vi "AMI_SetVoltage.vi"(6 "error in (no error)":errorcluster, 7 "Index":i8) -> (0 "error out":errorcluster, 2 "resulting string 1":string="        Set Temperatura 4.2K at 20K/min, FastSettle", 3 "Cancelled?":bool)   [LabVIEW 2017]
doc: "Use this template to create a dialog box. This template polls the state of the buttons on the front panel and does not use events. Use the Dialog Using Events template (not available in Base package) to create a dialog box with event handling."
panel:
  in  "Wait stability":bool=TRUE
  in  "Rate (V/min)":dbl=20.0
  in  "Voltage (V)":dbl=5.0
  in  "Cancel":bool
  in  "OK":bool
  # "SET VOLTAGE"
  # "Enero 2023 V1.3  a-sslcdms"
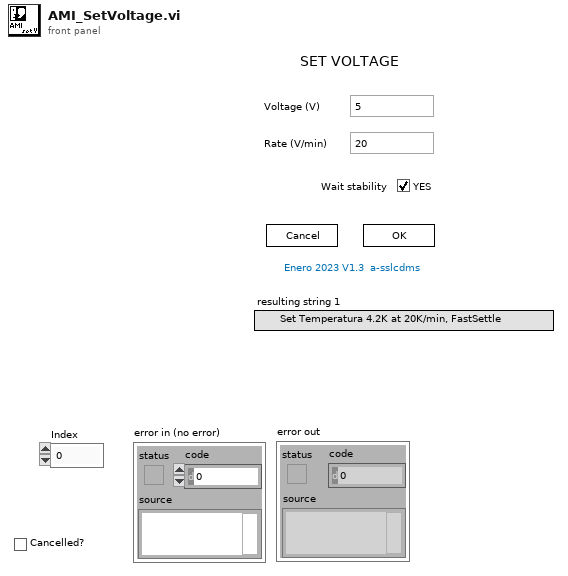
[diagram p1: front panel]
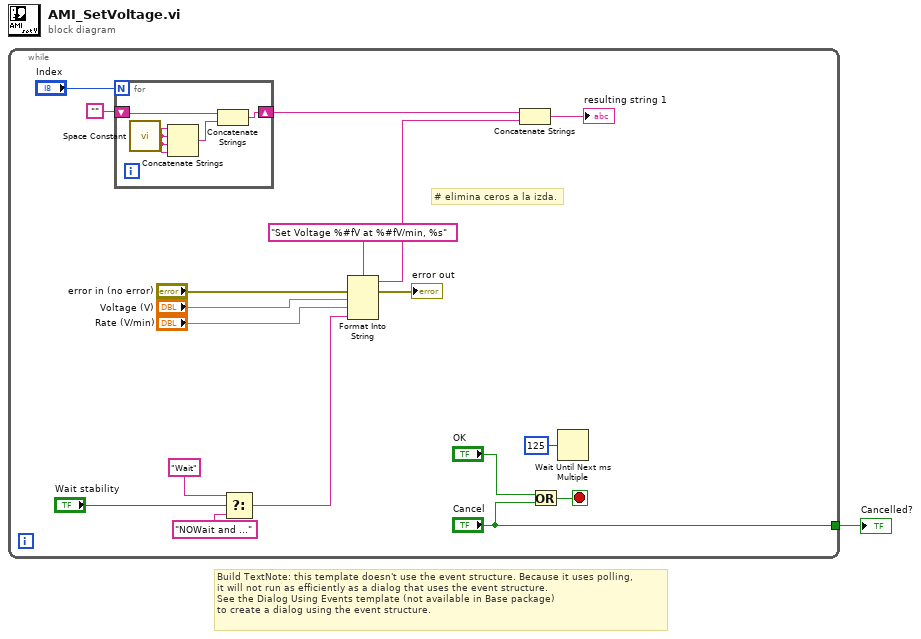
[diagram p0: block diagram]
diagram:
  # "Build TextNote: this template doesn't use the event structure. Because it uses polling, \nit will not run as efficiently as a dialog that uses the event structure.\nSee the Dialog Using Events template (not available in Base package) \nto create a dialog using the event structure."
  n1 = while {
    tunnel: ["Cancel"] -> w1
    stop <- w18 stop-if-true
    # "# elimina ceros a la izda."
    n2 = for {
      N: "Index" -> [_]
      shift-right: [w22] -> w8
      shift-left: "" -> [w21]
      n3 = call <vilib>:"Space Constant.vi"() -> ("String"=w20:string)
      n4 = Concatenate Strings(w20, w20, w20, w20) -> (w23:string)
      n5 = Concatenate Strings(w21, w23) -> (w22:string)
    }
    n6 = Select(t="Wait", s="Wait stability", f="NOWait and ...") -> (s? t:f=w2:string)
    n7 = Format Into String(format string="Set Voltage %#fV at %#fV/min, %s", error in="error in (no error)", "Voltage (V)", "Rate (V/min)", w2) -> (resulting string=w10:string, error out=→"error out":errorcluster)  [unwired: 1 in]
    n8 = Concatenate Strings(w8, w10) -> (→"resulting string 1":string)
    n9 = Or(x="OK", y="Cancel") -> (x .or. y?=w18:bool)
    n10 = Wait Until Next ms Multiple(millisecond multiple=u32 125) -> ()  [unwired: 1 out]
  }
  "Cancelled?" <- w1
